vi "Flow Compute.vi"(8 "error in":errorcluster, 11 "DAC FTCU in":refnum<class "DAC FTCU.lvclass">) -> (0 "error out":errorcluster, 1 "Status":map{string, bool}(c390), 2 "Flow":sgl, 3 "DAC FTCU out":refnum<class "DAC FTCU.lvclass">)   [LabVIEW 2019, in "DAC.lvlib" / "DAC FTCU.lvclass"]
uses:
  DAC FTCU.lvclass
  DAC FTCU.lvclass/DAC FTCU.ctl
  <vilib>/NI/Modbus Library/API/Master/Modbus Master.lvclass
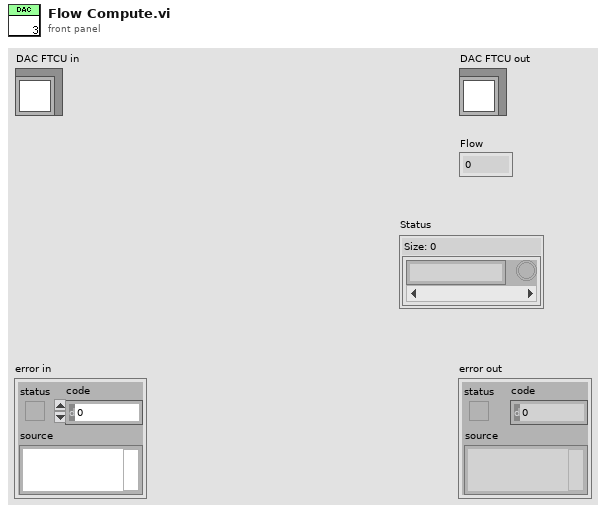
[diagram p1: front panel]
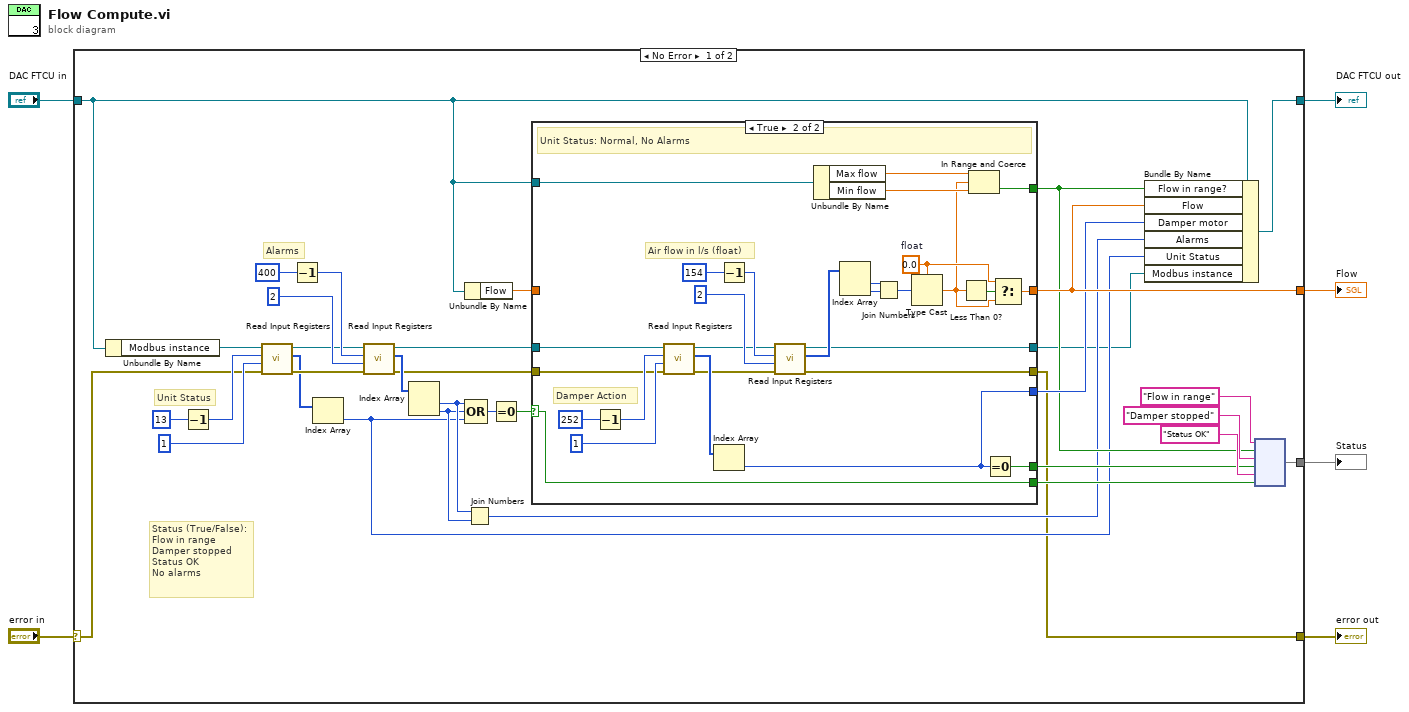
[diagram p0: block diagram]
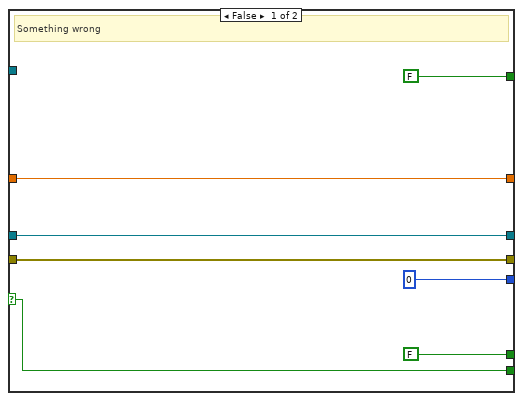
[diagram p2: hidden frame]
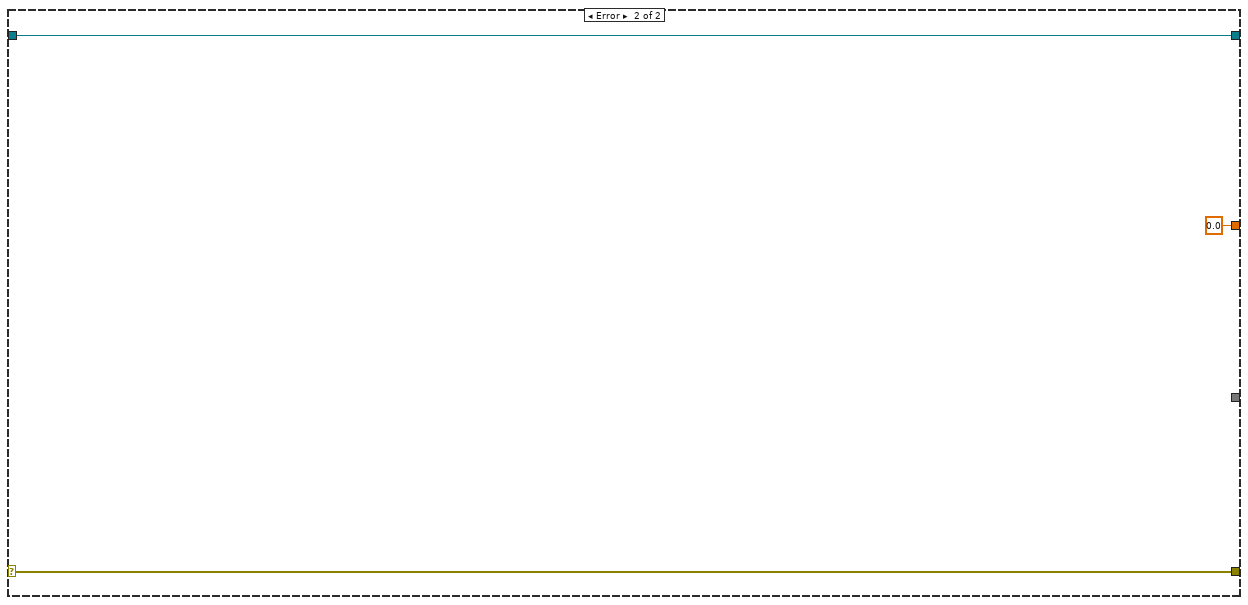
[diagram p3: hidden frame]
diagram:
  n1 = case shown="No Error" "error in" {
    selector: "error in" -> [w36 w78]
    tunnel: [w7 w78] -> w5
    tunnel: [w23 w77] -> w3
    tunnel: "DAC FTCU in" -> [w24 w77]
    tunnel: [w22 sgl 0.0 ("float")] -> w2
    tunnel: [w12 _] -> w1
    frame No Error {
      # "Alarms"
      # "Unit Status"
      # "Status (True/False):\nFlow in range\nDamper stopped\nStatus OK\nNo alarms"
      n2 = Unbundle By Name(w24) -> ("Modbus instance"=w37:refnum<class "Modbus Master.lvclass">)
      n3 = Decrement(x=u16 13 ("number of inputs")) -> (x-1=w39:u16)
      n4 = call-dynamic "Read Input Registers.vi"("error in"=w36, "number of inputs"=u16 1, "starting address"=w39, "Modbus master in"=w37) -> ("error out"=w31:errorcluster, "register values"=w30:u16[], "Modbus master out"=w32:refnum<class "Modbus Master.lvclass">)  [unwired: 5 in]
      n5 = Decrement(x=u16 400 ("number of inputs")) -> (x-1=w34:u16)
      n6 = Index Array(array=w30) -> (element=w9:u16)  [unwired: 1 in]
      n7 = call-dynamic "Read Input Registers.vi"("error in"=w31, "number of inputs"=u16 2, "starting address"=w34, "Modbus master in"=w32) -> ("error out"=w26:errorcluster, "register values"=w29:u16[], "Modbus master out"=w27:refnum<class "Modbus Master.lvclass">)  [unwired: 5 in]
      n8 = Index Array(array=w29) -> (element #1=w20:u16, element #2=w19:u16)  [unwired: 2 in]
      n9 = Unbundle By Name(w24) -> ("Flow"=w25:sgl)
      n10 = Compound Arithmetic op=OR(w20, w19, w9) -> (w28:u16)
      n11 = Join Numbers(hi=w20, lo=w19) -> ((hi.lo)=w10:u32)
      n12 = Equal To 0?(x=w28) -> (x = 0?=w13:bool)
      n13 = case shown="True" w13 {
        selector: w13 -> [w43 w57]
        tunnel: w27 -> [w42 w53]
        tunnel: w26 -> [w41 w71]
        tunnel: w25 -> [w45 _]
        tunnel: w24 -> [_ w70]
        tunnel: [w45 w50] -> w22
        tunnel: [FALSE w69] -> w15
        tunnel: [u16 0 ("register") w68] -> w21
        tunnel: [FALSE w67] -> w14
        tunnel: [w43 w57] -> w11
        tunnel: [w42 w56] -> w8
        tunnel: [w41 w54] -> w7
        frame False {
          # "Something wrong"
        }
        frame True {
          w49 = sgl 0.0  # float
          # "Air flow in l/s (float)"
          # "Damper Action"
          # "Unit Status: Normal, No Alarms"
          n14 = Decrement(x=u16 252 ("number of inputs")) -> (x-1=w73:u16)
          n15 = call-dynamic "Read Input Registers.vi"("error in"=w71, "number of inputs"=u16 1, "starting address"=w73, "Modbus master in"=w53) -> ("error out"=w55:errorcluster, "register values"=w75:u16[], "Modbus master out"=w52:refnum<class "Modbus Master.lvclass">)  [unwired: 5 in]
          n16 = Index Array(array=w75) -> (element=w68:u16)  [unwired: 1 in]
          n17 = Decrement(x=u16 154 ("number of inputs")) -> (x-1=w65:u16)
          n18 = call-dynamic "Read Input Registers.vi"("error in"=w55, "number of inputs"=u16 2, "starting address"=w65, "Modbus master in"=w52) -> ("error out"=w54:errorcluster, "register values"=w60:u16[], "Modbus master out"=w56:refnum<class "Modbus Master.lvclass">)  [unwired: 5 in]
          n19 = Unbundle By Name(w70) -> ("Max flow"=w59:sgl, "Min flow"=w58:sgl)
          n20 = Index Array(array=w60) -> (element #1=w64:u16, element #2=w63:u16)  [unwired: 2 in]
          n21 = Join Numbers(hi=w64, lo=w63) -> ((hi.lo)=w62:u32)
          n22 = Type Cast(type=w49, x=w62) -> (*(type *) &x=w48:sgl)
          n23 = Less Than 0?(x=w48) -> (x < 0?=w51:bool)
          n24 = In Range and Coerce(upper limit=w59, x=w48, lower limit=w58) -> (In Range?=w69:bool)  [unwired: 1 out]
          n25 = Equal To 0?(x=w68) -> (x = 0?=w67:bool)
          n26 = Select(t=w49, s=w51, f=w48) -> (s? t:f=w50:sgl)
        }
      }
      n27 = Bundle By Name(cluster=w24, "Flow in range?"=w15, "Flow"=w22, "Damper motor"=w21, "Alarms"=w10, "Unit Status"=w9, "Modbus instance"=w8) -> (w23:refnum<class "DAC FTCU.lvclass">)
      n28 = node("Flow in range" ("key"), w15, "Damper stopped" ("key"), w14, "Status OK" ("key"), w11) -> (w12:map{string, bool})
    }
    frame Error {
    }
  }
  "error out" <- w5
  "DAC FTCU out" <- w3
  "Status" <- w1
  "Flow" <- w2
